vi "SharedFileInf.vi"(1 "Write?":bool, 2 "FileInfInput":cluster{"Error in":T1, "File Handle in":u8} {"Error in" items=["SUCCESS"=0, "NO_HANDLES"=33024, "NO_FILES"=33536, "PARTIAL_WRITE"=33792, "EOF"=34048, "FILE_NOT_FOUND"=34560, "FILE_CLOSED"=34816, "NO_LINEAR_SPACE"=35072, "GENERIC_ERROR"=35328, "FILE_BUSY"=35584, "NO_WRITE_BUFFERS"=35840, "ILLEGAL_APPEND"=36096, "FILE_FULL"=36352, "FILE_EXISTS"=36608, "ILLEGAL_FILE_NAME"=37376, "ILLEGAL_HANDLE"=37632]}) -> (0 "FileInf":cluster{"Error in":T1, "File Handle in":u8} {"Error in" items=["SUCCESS"=0, "NO_HANDLES"=33024, "NO_FILES"=33536, "PARTIAL_WRITE"=33792, "EOF"=34048, "FILE_NOT_FOUND"=34560, "FILE_CLOSED"=34816, "NO_LINEAR_SPACE"=35072, "GENERIC_ERROR"=35328, "FILE_BUSY"=35584, "NO_WRITE_BUFFERS"=35840, "ILLEGAL_APPEND"=36096, "FILE_FULL"=36352, "FILE_EXISTS"=36608, "ILLEGAL_FILE_NAME"=37376, "ILLEGAL_HANDLE"=37632]})   [LabVIEW 2010, in "Player.lvlib"]
uses:
  Player.lvlib
  <vilib>/NXT/Block Support/NXT_FileStatusCodes.ctl
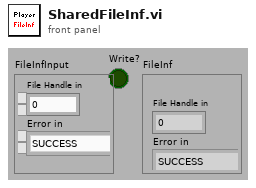
[diagram p1: front panel]
types:
  T1 = typedef "NXT_FileStatusCodes.ctl" = u16
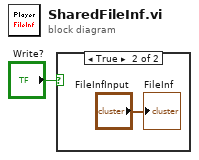
[diagram p0: block diagram]
diagram:
  n1 = case shown="True" "Write?" {
    frame False {
    }
    frame True {
      "FileInf" <- "FileInfInput"
    }
  }
